vi "Update Build Version.vi"(8 "error in (no error)":errorcluster, 11 "PostBuildSupport in":refnum<class "PostBuildSupport.lvclass">) -> (0 "error out":errorcluster, 3 "PostBuildSupport out":refnum<class "PostBuildSupport.lvclass">)   [LabVIEW 2016, in "PostBuildSupport.lvclass"]
uses:
  PostBuildSupport.lvclass
  <vilib>/AppBuilder/AB_API_Simple/Build Specification Version.ctl
  PostBuildSupport.lvclass/PostBuildSupport.ctl
  <vilib>/AppBuilder/AB_API_Simple/Set Build Specification Version (path).vi
  <vilib>/AppBuilder/AB_API_Simple/NI_App_Builder_API.lvlib
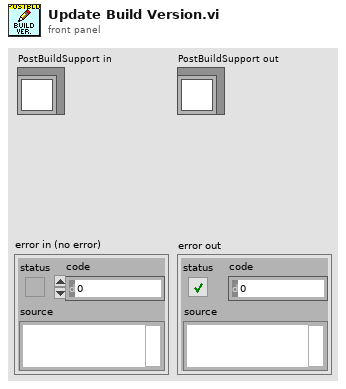
[diagram p1: front panel]
types:
  T1 = typedef "NI_App_Builder_API.lvlib/Build Specification Version.ctl" = cluster{"Major":u16, "Minor":u16, "Fix":u16, "Build":u16}
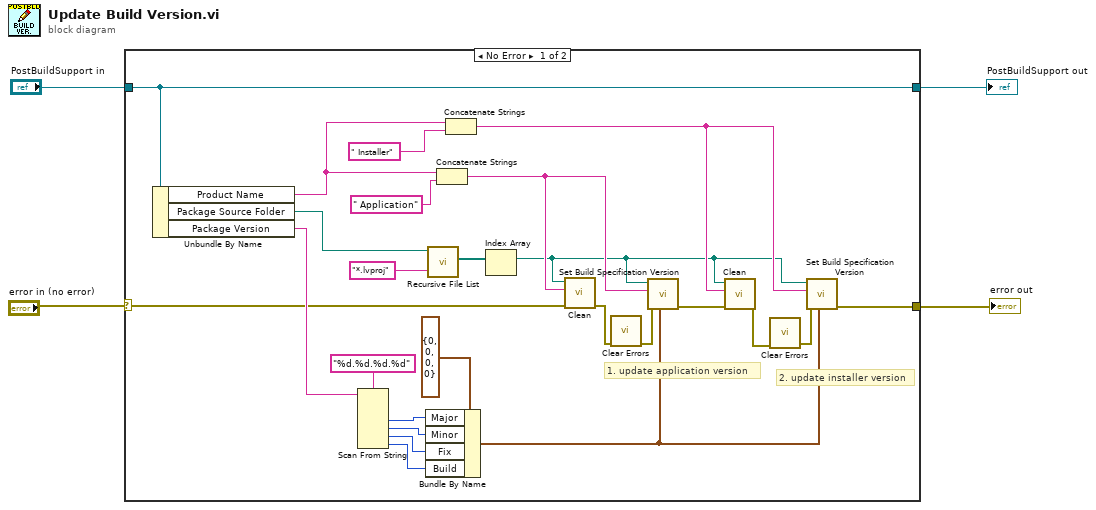
[diagram p0: block diagram]
diagram:
  n1 = case shown="No Error" "error in (no error)" {
    selector: "error in (no error)" -> [w9 w30]
    tunnel: [w29 w30] -> w4
    tunnel: "PostBuildSupport in" -> [w10 w31]
    tunnel: [w10 w31] -> w2
    frame No Error {
      # "2. update installer version"
      # "1. update application version"
      n2 = Unbundle By Name(w10) -> ("Product Name"=w12:string, "Package Source Folder"=w13:path, "Package Version"=w11:string)
      n3 = Scan From String(format string="%d.%d.%d.%d", input string=w11) -> (output 1=w24:i32, output 2=w27:i32, output 3=w23:i32, output 4=w26:i32)  [unwired: 6 in, 3 out]
      n4 = Bundle By Name(cluster=T1 {"Major"=0, "Minor"=0, "Fix"=0, "Build"=0} ("Build Specification Version"), "Major"=w24, "Minor"=w27, "Fix"=w23, "Build"=w26) -> (w28:T1)
      n5 = call <vilib>:"Recursive File List.vi"("pattern"="*.lvproj", "Folder Path"=w13) -> ("All Files in Dir"=w15:path[])  [unwired: 5 in, 4 out]
      n6 = Concatenate Strings(w12, " Application" ("Name of target (My Computer)")) -> (w19:string)
      n7 = Concatenate Strings(w12, " Installer" ("Name of target (My Computer)")) -> (w17:string)
      n8 = Index Array(array=w15) -> (element=w14:path)  [unwired: 1 in]
      n9 = call <vilib>:"Clean.vi"("error in (no error)"=w9, "Name of build specification (if empty: clean all)"=w19, "Path to project"=w14) -> ("error out"=w8:errorcluster)  [unwired: 8 in]
      n10 = call <vilib>:"Clear Errors.vi"("error in (no error)"=w8) -> ("error out"=w7:errorcluster)  [unwired: 5 in, 1 out]
      n11 = call-poly <vilib>:"Set Build Specification Version.vi"("Build Specification Version"=w28, "error in (no error)"=w7, "Name of build specification"=w19, "Path to project"=w14) -> ("error out"=w21:errorcluster)  [unwired: 7 in]
      n12 = call <vilib>:"Clean.vi"("error in (no error)"=w21, "Name of build specification (if empty: clean all)"=w17, "Path to project"=w14) -> ("error out"=w6:errorcluster)  [unwired: 8 in]
      n13 = call <vilib>:"Clear Errors.vi"("error in (no error)"=w6) -> ("error out"=w5:errorcluster)  [unwired: 5 in, 1 out]
      n14 = call-poly <vilib>:"Set Build Specification Version.vi"("Build Specification Version"=w28, "error in (no error)"=w5, "Name of build specification"=w17, "Path to project"=w14) -> ("error out"=w29:errorcluster)  [unwired: 7 in]
    }
    frame Error {
    }
  }
  "error out" <- w4
  "PostBuildSupport out" <- w2
